vi "Write outputs.vi"(5 "outputs":refnum<class "Terminal.lvclass">[](array[class]), 9 "FlatSequence in":refnum<class "FlatSequence.lvclass">) -> (3 "FlatSequence out":refnum<class "FlatSequence.lvclass">)   [LabVIEW 2014, in "FlatSequence.lvclass"]
uses:
  FlatSequence.lvclass
  Terminal/Terminal.lvclass
  FlatSequence.lvclass/FlatSequence.ctl
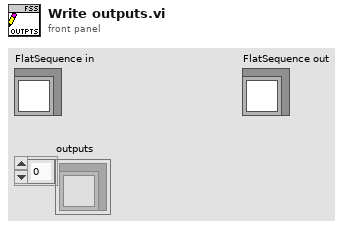
[diagram p1: front panel]
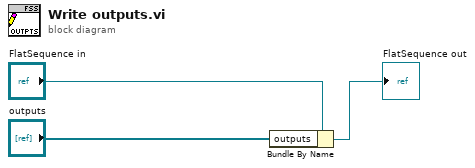
[diagram p0: block diagram]
diagram:
  n1 = Bundle By Name(cluster="FlatSequence in", "outputs"="outputs") -> (→"FlatSequence out":refnum<class "FlatSequence.lvclass">)
